vi "Build Exp Wvfrm (Cluster).vi"(8 "error in (no error)":errorcluster, 9 "Express Waveform Attributes":T1 {"Timestamp" format="%<%X\n%x>T"; "Start Timestamp" format="%<%X\n%x>T"}, 11 "Signal Components":cluster{"X0":dbl, "dX":dbl, "Y":dbl[]} {"Y" format="%0.2f"; "dX" format="%0.6f"; "X0" format="%0.6f"}) -> (0 "error out":errorcluster, 3 "Waveform":waveform(dbl))   [LabVIEW 2017]
uses:
  <vilib>/express/express shared/transition.llb/ex_WaveformAttribs.ctl
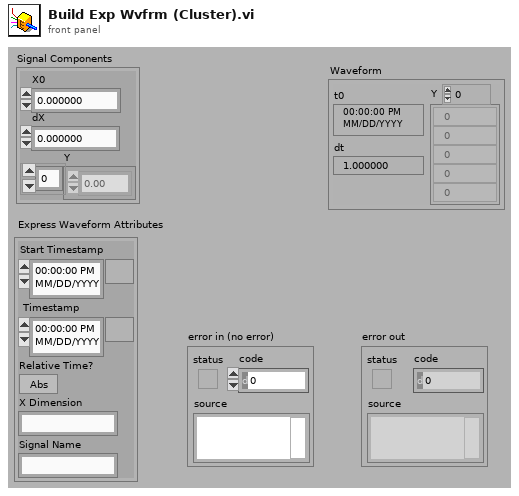
[diagram p1: front panel]
types:
  T1 = typedef "ex_WaveformAttribs.ctl" = cluster{"Start Timestamp":timestamp, "Timestamp":timestamp, "Relative Time?":bool, "X Dimension":string, "Signal Name":string}
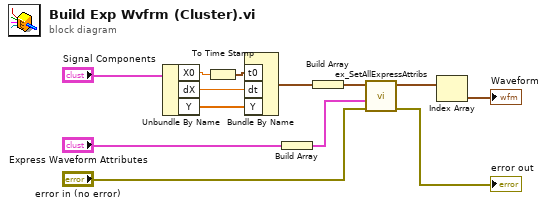
[diagram p0: block diagram]
diagram:
  n1 = Unbundle By Name("Signal Components") -> ("X0"=w10:dbl, "dX"=w9:dbl, "Y"=w8:dbl[])
  n2 = To Time Stamp(1:w10) -> (0:w1:timestamp)
  n3 = Bundle By Name("t0"=w1, "dt"=w9, "Y"=w8) -> (w12:waveform(dbl))  [unwired: 1 in]
  n4 = Build Array("Express Waveform Attributes") -> (w7:T1[])
  n5 = Build Array(w12) -> (w6:waveform(dbl)[])
  n6 = call <vilib>:"ex_SetAllExpressAttribs.vi"("error in"="error in (no error)", "All Express Wave Attributes"=w7, "Signals"=w6) -> ("error out"=→"error out":errorcluster, "Signals With Attributes"=w5:waveform(dbl)[])  [unwired: 7 in]
  n7 = Index Array(array=w5) -> (element=→"Waveform":waveform(dbl))  [unwired: 1 in]
